vi "Create Time Entry.vi"(8 "error in (no error)":errorcluster, 9 "Task":string, 10 "Project":string, 11 "Time Entries in":refnum<class "Time Entries.lvclass">) -> (0 "error out":errorcluster, 2 "Initial Display":string[](array[string]), 3 "Time Entries out":refnum<class "Time Entries.lvclass">)   [LabVIEW 2020, in "Time Entries.lvclass"]
uses:
  Time Entries.lvclass
  Time Entries.lvclass/Time Entries.ctl
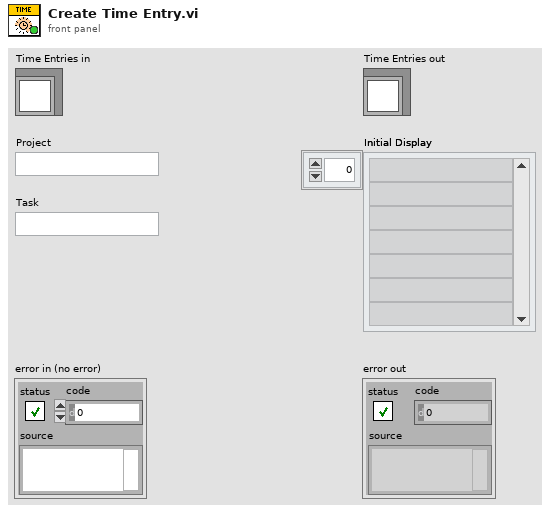
[diagram p1: front panel]
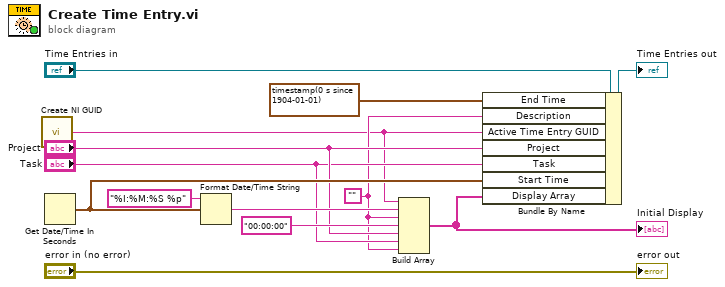
[diagram p0: block diagram]
diagram:
  w4 = ""
  n1 = call <vilib>:"Create NI GUID.vi"() -> ("NI GUID"=w1:string)
  n2 = Get Date/Time In Seconds() -> (seconds since 1Jan1904=w10:timestamp)
  n3 = Format Date/Time String(time format string (%c)="%I:%M:%S %p", seconds (now)=w10) -> (date/time string=w8:string)  [unwired: 1 in]
  n4 = Build Array(w1, w8, w4, "00:00:00" ("element"), "Project", "Task", w4) -> (w2:string[])
  "Initial Display" <- w2
  n5 = Bundle By Name(cluster="Time Entries in", "End Time"=timestamp(0 s since 1904-01-01), "Description"=w4, "Active Time Entry GUID"=w1, "Project"="Project", "Task"="Task", "Start Time"=w10, "Display Array"=w2) -> (→"Time Entries out":refnum<class "Time Entries.lvclass">)
  "error out" <- "error in (no error)"
